vi "To CSV File.vi"(8 "error in (no error)":errorcluster, 9 "Path":path, 10 "engine configuration":refnum<class "engine configuration.lvclass">, 11 "J1939 editor node in":refnum<class "J1939 editor node.lvclass">) -> (0 "error out":errorcluster, 3 "J1939 editor node out":refnum<class "J1939 editor node.lvclass">)   [LabVIEW 2017, in "J1939 editor node.lvclass"]
uses:
  J1939 editor node.lvclass
  <vilib>/NI/Module Execution Interface/Engine Configuration/engine configuration.lvclass
  module/configuration/J1939 configuration.lvclass
  C:/Program Files (x86)/National Instruments/LabVIEW 2017/vi.lib/NI/Configuration Framework/serializable configuration/NISE_CEF_serializable configuration.lvclass
  <vilib>/NI/Configuration Framework/serializable configuration/NISE_CEF_serializable configuration.lvclass/NISE_CEF_serializable configuration.ctl
  module/configuration/J1939 configuration.lvclass/J1939 configuration.ctl
  <vilib>/NI/Tag Bus/tag/tag descriptor.lvclass/tag descriptor.ctl
  <vilib>/Utility/LVClass/Get LV Class Name.vi
  <vilib>/NI/Configuration Framework/error generator/NISE_error generator.vi
  <vilib>/Utility/file.llb/Write Delimited Spreadsheet (string).vi
  <vilib>/NI/Tag Bus Module Framework/channel/TBM channel.lvclass
  <vilib>/NI/Configuration Framework/serializable configuration/NISE_CEF_serializable configuration.lvclass
  <vilib>/NI/Tag Bus/tag/tag descriptor.lvclass
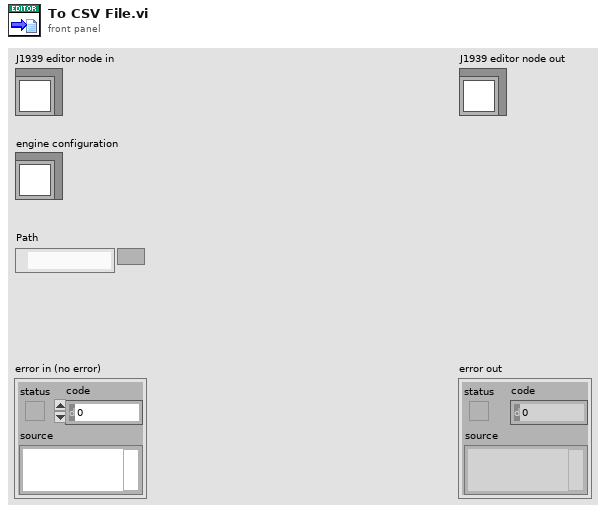
[diagram p1: front panel]
types:
  T1 = typedef "J1939 configuration.lvclass/Line.ctl" = cluster{"channel":refnum<class "TBM channel.lvclass">, "XNET Signal":refnum<k21>}
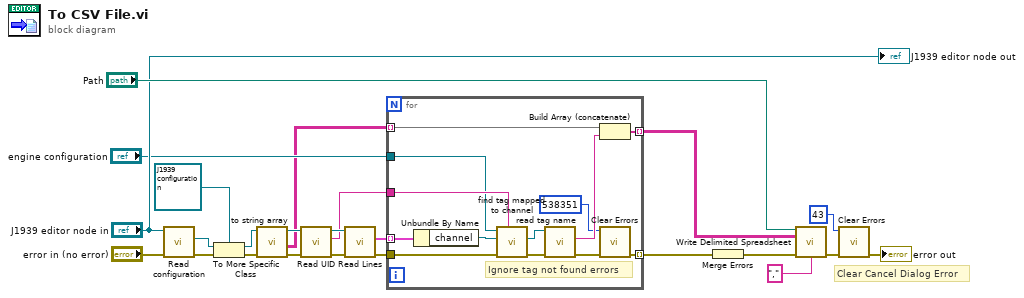
[diagram p0: block diagram]
diagram:
  # "Clear Cancel Dialog Error"
  n1 = call-dynamic "Read configuration.vi"("error in"="error in (no error)", "J1939 editor node in"="J1939 editor node in") -> ("error out"=w19:errorcluster, "configuration"=w18:refnum<class "NISE_CEF_serializable configuration.lvclass">)  [unwired: 7 in, 1 out]
  n2 = To More Specific Class(target class=refnum<class "J1939 configuration.lvclass"> refnum ("J1939 configuration"), reference=w18, error in=w19) -> (specific class reference=w15:refnum<class "J1939 configuration.lvclass">, error out=w16:errorcluster)
  n3 = call-dynamic "to string array.vi"("error in (no error)"=w16, "module configuration in"=w15) -> ("error out"=w14:errorcluster, "Array"=w9:string[][], "module configuration out"=w12:refnum<class "J1939 configuration.lvclass">)  [unwired: 6 in, 1 out]
  n4 = call <vilib>:"Read UID.vi"("error in"=w14, "configuration in"=w12) -> ("error out"=w13:errorcluster, "instance id"=w8:string, "configuration out"=w11:refnum<class "J1939 configuration.lvclass">)  [unwired: 7 in]
  n5 = call "Read Lines.vi"("error in (no error)"=w13, "J1939 configuration in"=w11) -> ("error out"=w1:errorcluster, "Lines"=w10:T1[])  [unwired: 7 in, 1 out]
  n6 = for {
    tunnel: w10 -> [w37] mode=indexing
    tunnel: w9 -> [w33] mode=indexing
    tunnel: w8 -> [w36]
    tunnel: "engine configuration" -> [w34]
    tunnel: [w30] -> w7 mode=indexing
    tunnel: [w26] -> w3 mode=indexing
    tunnel: w1 -> [w25]
    # "Ignore tag not found errors"
    n7 = Unbundle By Name(w37) -> ("channel"=w35:refnum<class "TBM channel.lvclass">)
    n8 = call <vilib>:"find tag mapped to channel.vi"("owner"=w36, "error in"=w25, "channel"=w35, "engine configuration in"=w34) -> ("error out"=w29:errorcluster, "tag"=w32:refnum<class "tag descriptor.lvclass">)  [unwired: 5 in, 1 out]
    n9 = call <vilib>:"read tag name.vi"("error in"=w29, "system tag in"=w32) -> ("error out"=w27:errorcluster, "name"=w31:string)  [unwired: 7 in, 1 out]
    n10 = Build Array (concatenate)(w33, w31) -> (w30:string[])
    n11 = call <vilib>:"Clear Errors.vi"("error in (no error)"=w27, "specific error code to clear (0: all)"=538351) -> ("error out"=w26:errorcluster)  [unwired: 4 in, 1 out]
  }
  n12 = Merge Errors(w3) -> (w2:errorcluster)
  n13 = call-poly <vilib>:"Write Delimited Spreadsheet.vi"("file path (dialog if empty)"="Path", "2D data"=w7, "error in (no error)"=w2, "delimiter (\\t)"="," ("delimiter (\\t)")) -> ("error out"=w4:errorcluster)  [unwired: 10 in, 1 out]
  n14 = call <vilib>:"Clear Errors.vi"("error in (no error)"=w4, "specific error code to clear (0: all)"=43) -> ("error out"=→"error out":errorcluster)  [unwired: 4 in, 1 out]
  "J1939 editor node out" <- "J1939 editor node in"
